vi "Append Path to Current VIs Folder.vi"(8 "error in":errorcluster, 11 "name or relative path":path) -> (0 "error out":errorcluster, 3 "appended path":path)   [LabVIEW 2025]
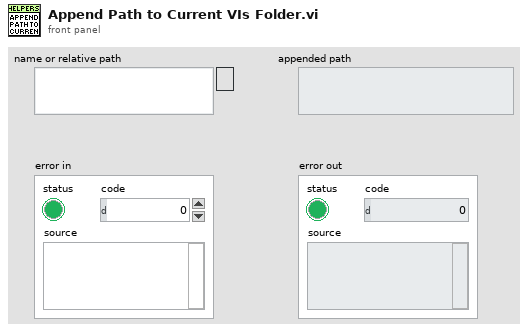
[diagram p1: front panel]
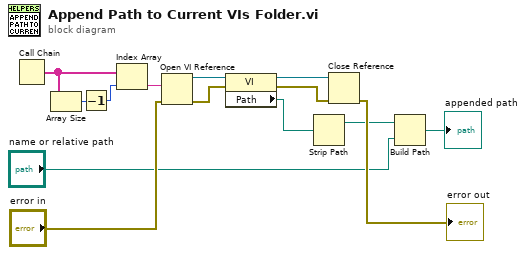
[diagram p0: block diagram]
diagram:
  n1 = Call Chain() -> (call chain=w10:string[])
  n2 = Array Size(array=w10) -> (size(s)=w11:i32)
  n3 = Decrement(x=w11) -> (x-1=w12:i32)
  n4 = Index Array(array=w10, index=w12) -> (element=w13:string)
  n5 = Open VI Reference(vi path=w13, error in (no error)="error in") -> (vi reference=w14:refnum<vi>, error out=w7:errorcluster)  [unwired: 4 in]
  n6 = property class="VI"(reference=w14, error in=w7) -> (reference out=w9:refnum<vi>, error out=w6:errorcluster, "Path"=w4:path)
  n7 = Strip Path(path=w4) -> (stripped path=w3:path)  [unwired: 1 out]
  n8 = Close Reference(reference=w9, error in (no error)=w6) -> (error out=→"error out":errorcluster)
  n9 = Build Path(base path=w3, name or relative path="name or relative path") -> (appended path=→"appended path":path)
